vi "CC Get Device By Name.vi"(8 "error in (no error)":errorcluster, 11 "Device Type":string) -> (0 "error out":errorcluster, 2 "Hardware Config out":T1, 3 "Device":T2)   [LabVIEW 2021]
uses:
  typedefs/CC cluster Device Index.ctl
  typedefs/CC cluster Hardware Config.ctl
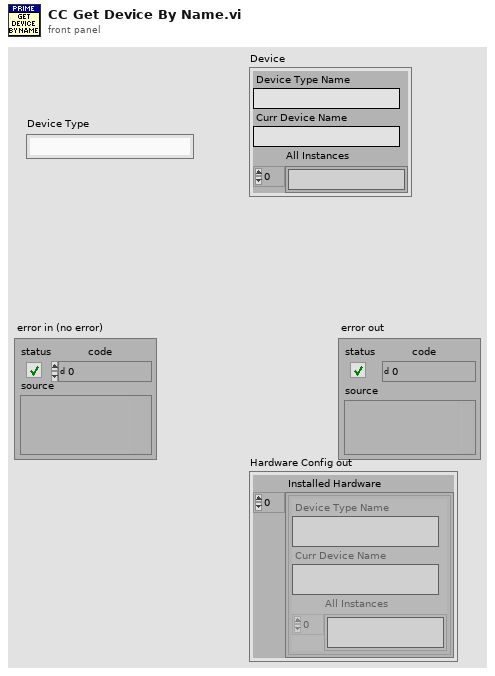
[diagram p1: front panel]
types:
  T1 = typedef "CC cluster Hardware Config.ctl" = cluster{"Installed Hardware":T2[]}
  T2 = typedef "CC cluster Device Index.ctl" = cluster{"Device Type Name":string, "Curr Device Name":string, "All Instances":string[]}
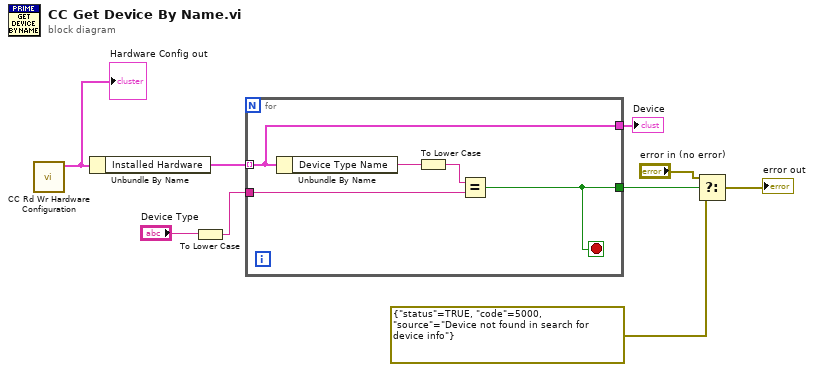
[diagram p0: block diagram]
diagram:
  n1 = call "CC Rd Wr Hardware Configuration.vi"() -> ("Hardware Config out"=w9:T1)  [unwired: 9 in, 2 out]
  "Hardware Config out" <- w9
  n2 = Unbundle By Name(w9) -> ("Installed Hardware"=w8:T2[])
  n3 = To Lower Case(string="Device Type") -> (all lower case string=w6:string)
  n4 = for {
    tunnel: w8 -> [w11] mode=indexing
    tunnel: w6 -> [w12]
    tunnel: [w11] -> w5
    tunnel: [w10] -> w4
    stop <- w10 stop-if-true
    n5 = Unbundle By Name(w11) -> ("Device Type Name"=w14:string)
    n6 = To Lower Case(string=w14) -> (all lower case string=w13:string)
    n7 = Equal?(x=w13, y=w12) -> (x = y?=w10:bool)
  }
  "Device" <- w5
  n8 = Select(t="error in (no error)", s=w4, f=errorcluster {"status"=TRUE, "code"=5000, "source"="Device not found in search for device info"}) -> (s? t:f=→"error out":errorcluster)
